vi "Read filter.vi"(8 "error in":errorcluster, 11 "CRDS Data in":refnum<class "CRDS Data.lvclass">) -> (0 "error out":errorcluster, 2 "filter":bool, 3 "CRDS Data out":refnum<class "CRDS Data.lvclass">)   [LabVIEW 2018, in "CRDS Lib.lvlib" / "CRDS Data.lvclass"]
doc: "Retrieve the current state of the filter associated with the CRDS sample line. True is filtered and false is sample."
uses:
  CRDS Data.lvclass
  CRDS Data.lvclass/CRDS Data.ctl
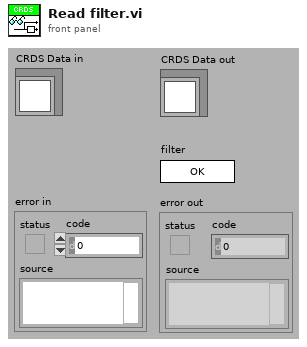
[diagram p1: front panel]
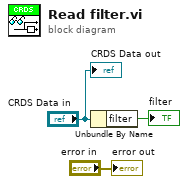
[diagram p0: block diagram]
diagram:
  n1 = Unbundle By Name("CRDS Data in") -> ("filter"=→"filter":bool)
  "error out" <- "error in"
  "CRDS Data out" <- "CRDS Data in"
